vi "Set_TargetFile_Name.vi"(7 "Target Operating System":T1(ring), 8 "error in (no error)":errorcluster, 9 "Target file type":T2, 10 "Target file name":string, 11 "AB_Targetfile in":refnum<class "AB_Targetfile.lvclass">) -> (0 "error out":errorcluster, 3 "AB_Targetfile out":refnum<class "AB_Targetfile.lvclass">)   [LabVIEW 2020, in "AB_Targetfile.lvclass"]
uses:
  <vilib>/AppBuilder/AB_Classes/TargetFile/AB_Targetfile.lvclass
  <vilib>/AppBuilder/AB_TargetFileType.ctl
  <vilib>/AppBuilder/AB_Classes/TargetFile/AB_Targetfile.lvclass/AB_Targetfile.ctl
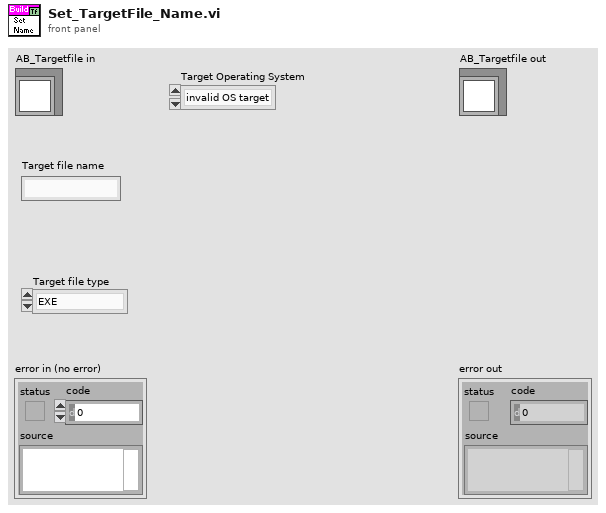
[diagram p1: front panel]
types:
  T1 = enum32{"invalid OS target", "Mac OS", "Windows 3.1", "Windows 95/NT", "Solaris 1", "Solaris 2", "HP-UX", "PowerMAX", "Linux", "Irix", "Rhapsody", "BeOS", "AIX", "OSF1", "VxWorks", "PharLap", "Carbon", "RTX", "Windows x64", "Linux x64", "Mac OS X x64"}
  T2 = typedef "AB_TargetFileType.ctl" = enum16{"EXE", "DLL", "RTEXE"}
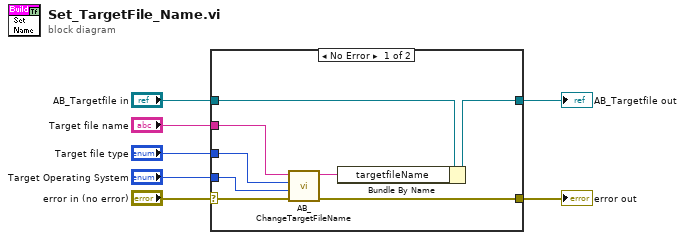
[diagram p0: block diagram]
diagram:
  n1 = case shown="No Error" "error in (no error)" {
    selector: "error in (no error)" -> [w9 w17]
    tunnel: [w13 w17] -> w6
    tunnel: [w14 w16] -> w4
    tunnel: "AB_Targetfile in" -> [w10 w16]
    tunnel: "Target file name" -> [w12 _]
    tunnel: "Target file type" -> [w11 _]
    tunnel: "Target Operating System" -> [w8 _]
    frame No Error {
      n2 = call <vilib>:"AB_ChangeTargetFileName.vi"("error in (no error)"=w9, "Target Operating System"=w8, "Build type"=w11, "Target file name"=w12) -> ("error out"=w13:errorcluster, "New target file name"=w15:string)  [unwired: 6 out]
      n3 = Bundle By Name(cluster=w10, "targetfileName"=w15) -> (w14:refnum<class "AB_Targetfile.lvclass">)
    }
    frame Error {
    }
  }
  "error out" <- w6
  "AB_Targetfile out" <- w4
